vi "AO Write.vi"(7 "AO line":T1=5100 items=["ModB/AO0"=5100, "ModB/AO1"=5101, "ModB/AO2"=5102, "ModB/AO3"=5103], 8 "error in (no error)":errorcluster, 10 "data":dbl, 11 "direct IO in":refnum<class "NI_Robotics_Starter Kit Direct IO.lvclass">) -> (0 "error out":errorcluster, 3 "direct IO out":refnum<class "NI_Robotics_Starter Kit Direct IO.lvclass">)   [LabVIEW 2017, in "NI_Robotics_Starter Kit Direct IO.lvclass"]
uses:
  <vilib>/robotics/Starter Kit/Direct IO/NI_Robotics_Starter Kit Direct IO.lvclass
  <vilib>/robotics/Starter Kit/Direct IO/AO Lines.ctl
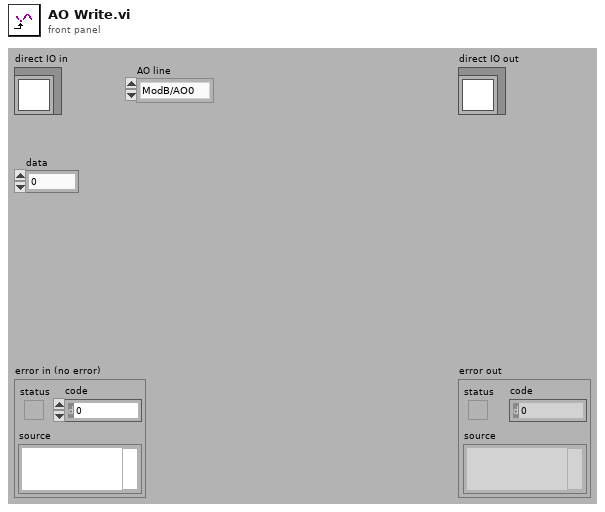
[diagram p1: front panel]
types:
  T1 = typedef "NI_Robotics_Starter Kit Direct IO.lvclass/AO Lines.ctl" = u16
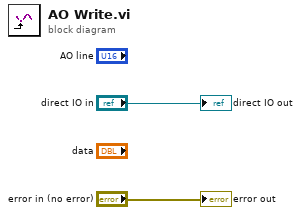
[diagram p0: block diagram]
diagram:
  "error out" <- "error in (no error)"
  "direct IO out" <- "direct IO in"
